vi "parse_string_scalar.vi"(4 "error in":errorcluster, 6 "type":string, 7 "msg in":string) -> (0 "error out":errorcluster, 2 "string":string, 3 "msg out":string)   [LabVIEW 2014]
doc: "Parses out a string array from msg in. The remaining string is returned in msg out."
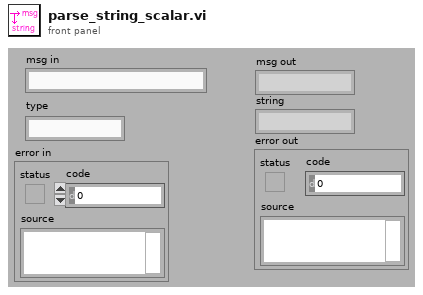
[diagram p1: front panel]
types:
  T1 = enum16{"big-endian, network order", "native, host order", "little-endian"}
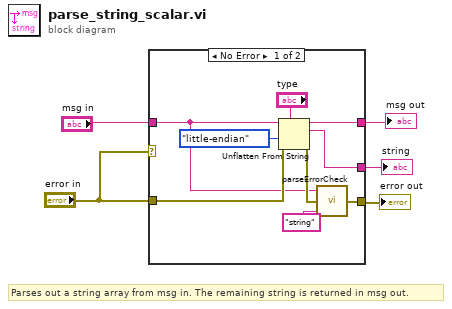
[diagram p0: block diagram]
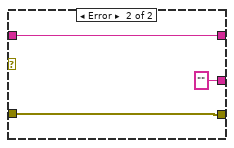
[diagram p2: hidden frame]
diagram:
  # "Parses out a string array from msg in. The remaining string is returned in msg out."
  n1 = case shown="No Error" "error in" {
    tunnel: "msg in" -> [w6 w17]
    tunnel: [w14 w17] -> w4
    tunnel: [w13 "" ("type")] -> w3
    tunnel: [w9 w15] -> w2
    tunnel: "error in" -> [w7 w15]
    frame No Error {
      n2 = Unflatten From String(type="type", binary string=w6, byte order (0:big-endian, network order)=T1."little-endian", error in (no error)=w7) -> (rest of the binary string=w14:string, value=w13:string, error out=w10:errorcluster)  [unwired: 1 in]
      n3 = call "parseErrorCheck.vi"("type"="string", "error in"=w10, "msg read"=w6) -> ("error out"=w9:errorcluster)
    }
    frame Error {
    }
  }
  "msg out" <- w4
  "string" <- w3
  "error out" <- w2
